vi "pco.camera_FloatingMean_Example_IMAQ.vi"() -> ()   [LabVIEW 2019]
uses:
  pco.camera/Camera.lvclass
  <vilib>/vision/NI_Vision_Development_Module.lvlib
panel:
  out "nominatorU64":u64 format="%x"
  out "denominatorU64":u64 format="%x"
  out "currentImage":T1(plugin-control)
  out "nominatorU32":u64 format="%x"
  out "denominatorU32":u64 format="%x"
  in  "averageCount":u8=10 caption="Average Count" min=2
  out "Image":T1(plugin-control)
  in  "data_format":T2(ring)=enum."Mono16"
  out "Recorded Images":u32
  in  "Quit":bool
  in  "roiY1":u64=2048 min=2 max=20000 step=1
  in  "roiX1":u64=2048 min=2 max=20000 step=1
  in  "roiY0":u64=1 min=1 max=1039 step=1
  in  "roiX0":u64=1 min=1 max=1391 step=1
  out "Image Height":u64
  out "Image Width":u64
  in  "dwImgCount":u32=10 caption="Fifo Buffer Size" max=4023
  out "Error":errorcluster {"code" format="%x"}
  # "This example shows how to compute and show a floating mean live image.\nHere the camera class is operated in fifo mode to always get next image in buffer.\nThe Average Count defines the number of images that will be averaged.\nAveraging is done by fetiching one image and using average image from previous iteration\n(avg_n = (1-1/avg_count)*avg_(n-1) + (1/avg_count)*image_n)\n\nIt is a good starting point for writing own applications.\nBut it will not be fail save, i.e. doesnt react on errors, just handles them forward to the end\n\nUsage:\nSelect your required fifo buffer size and image format and start the program.\nOnce started, the camera class will be initialized and image record will start automatically.\nInside the acquisition loop the program calculates the floating average image shows it.\nThe average count can be changed at any time.\nBy using the ROI parameters you can crop the image to select certain regions\n\nBy clicking Quit Application the record will stop and will force an exit of the camera class"
  # "pco.labview"
  # "Camera Setup"
  # "Recording Control"
  # "Parameters for image readout"
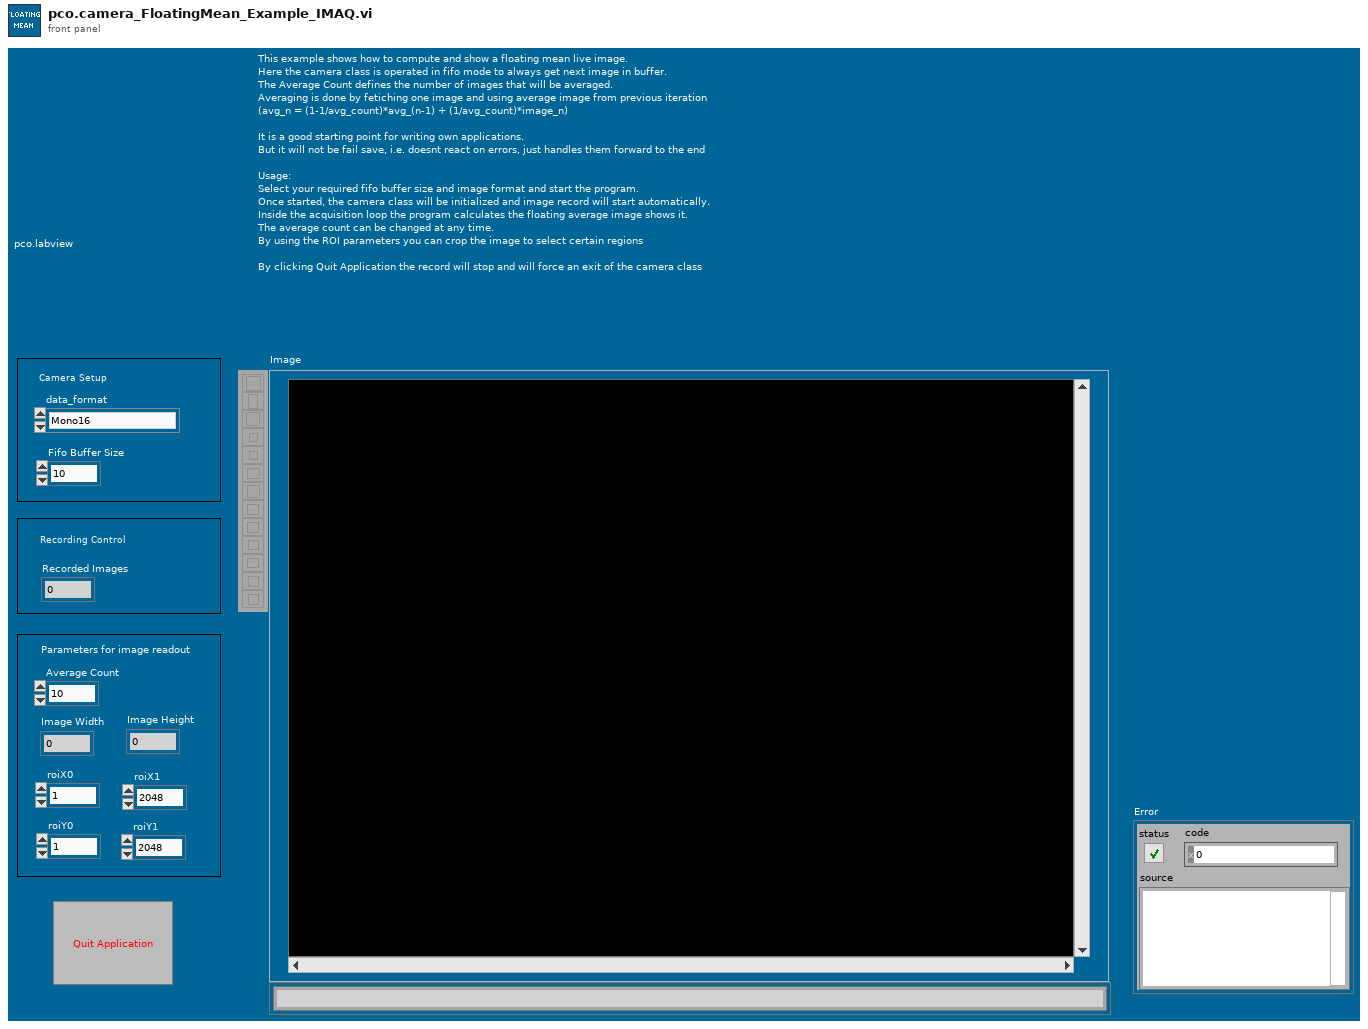
[diagram p1: front panel]
types:
  T1 = typedef "IMAQ Image.ctl" = refnum<image>
  T2 = enum16{"Undefined", "Mono8", "Mono16", "BGRA8", "RGBA8", "BGRA16", "RGBA16", "CompressedMono8"}
  T3 = enum8{"Enabled", "Disabled", "Disabled and Grayed Out"}
  T4 = enum16{"sequence", "sequence non blocking", "ring buffer", "fifo", "sequence_dpcore", "sequence_non_blocking_dpcore", "ring_buffer_dpcore", "fifo_dpcore", "tif", "multitif", "pcoraw", "b16", "dicom", "multidicom"}
  T5 = cluster{"serial":u32, "type":u16, "sub_type":u16, "interface_type":u16, "bit_resolution":u16, "min_exposure_time_s":dbl, "max_exposure_time_s":dbl, "min_exposure_step_s":dbl, "min_delay_time_s":dbl, "max_delay_time_s":dbl, "min_delay_step_s":dbl, "min_width":u64, "min_height":u64, "max_width":u64, "max_height":u64, "roi_step_horz":u64, "roi_step_vert":u64, "roi_symmetric_horz":bool, "roi_symmetric_vert":bool, "has_timestamp_mode":bool, "has_timestamp_mode_ascii_only":bool, "pixelrate_vec":u32[], "has_acquire_mode":bool, "has_ext_acquire_mode":bool, "has_metadata_mode":bool, "has_ram":bool, "binning_horz_vec":u16[], "binning_vert_vec":u16[]}
  T6 = typedef "Image Type" = u32
  T7 = typedef "Camera.lvclass/binning.ctl" = cluster{"vert":u16, "horz":u16}
  T8 = cluster{"exposure_time_s":dbl, "delay_time_s":dbl, "roi":cluster{"x0":u64, "y0":u64, "x1":u64, "y1":u64}, "timestamp_mode":u16, "pixelrate":u32, "trigger_mode":u16, "acquire_mode":u16, "metadata_mode":u16, "noisefilter_mode":u16, "binning":T7}
  T9 = cluster{"Plane 4 (alpha)":u16, "Plane 1 (Red)":u16, "Plane 2 (Green)":u16, "Plane 3 (Blue)":u16}[][]
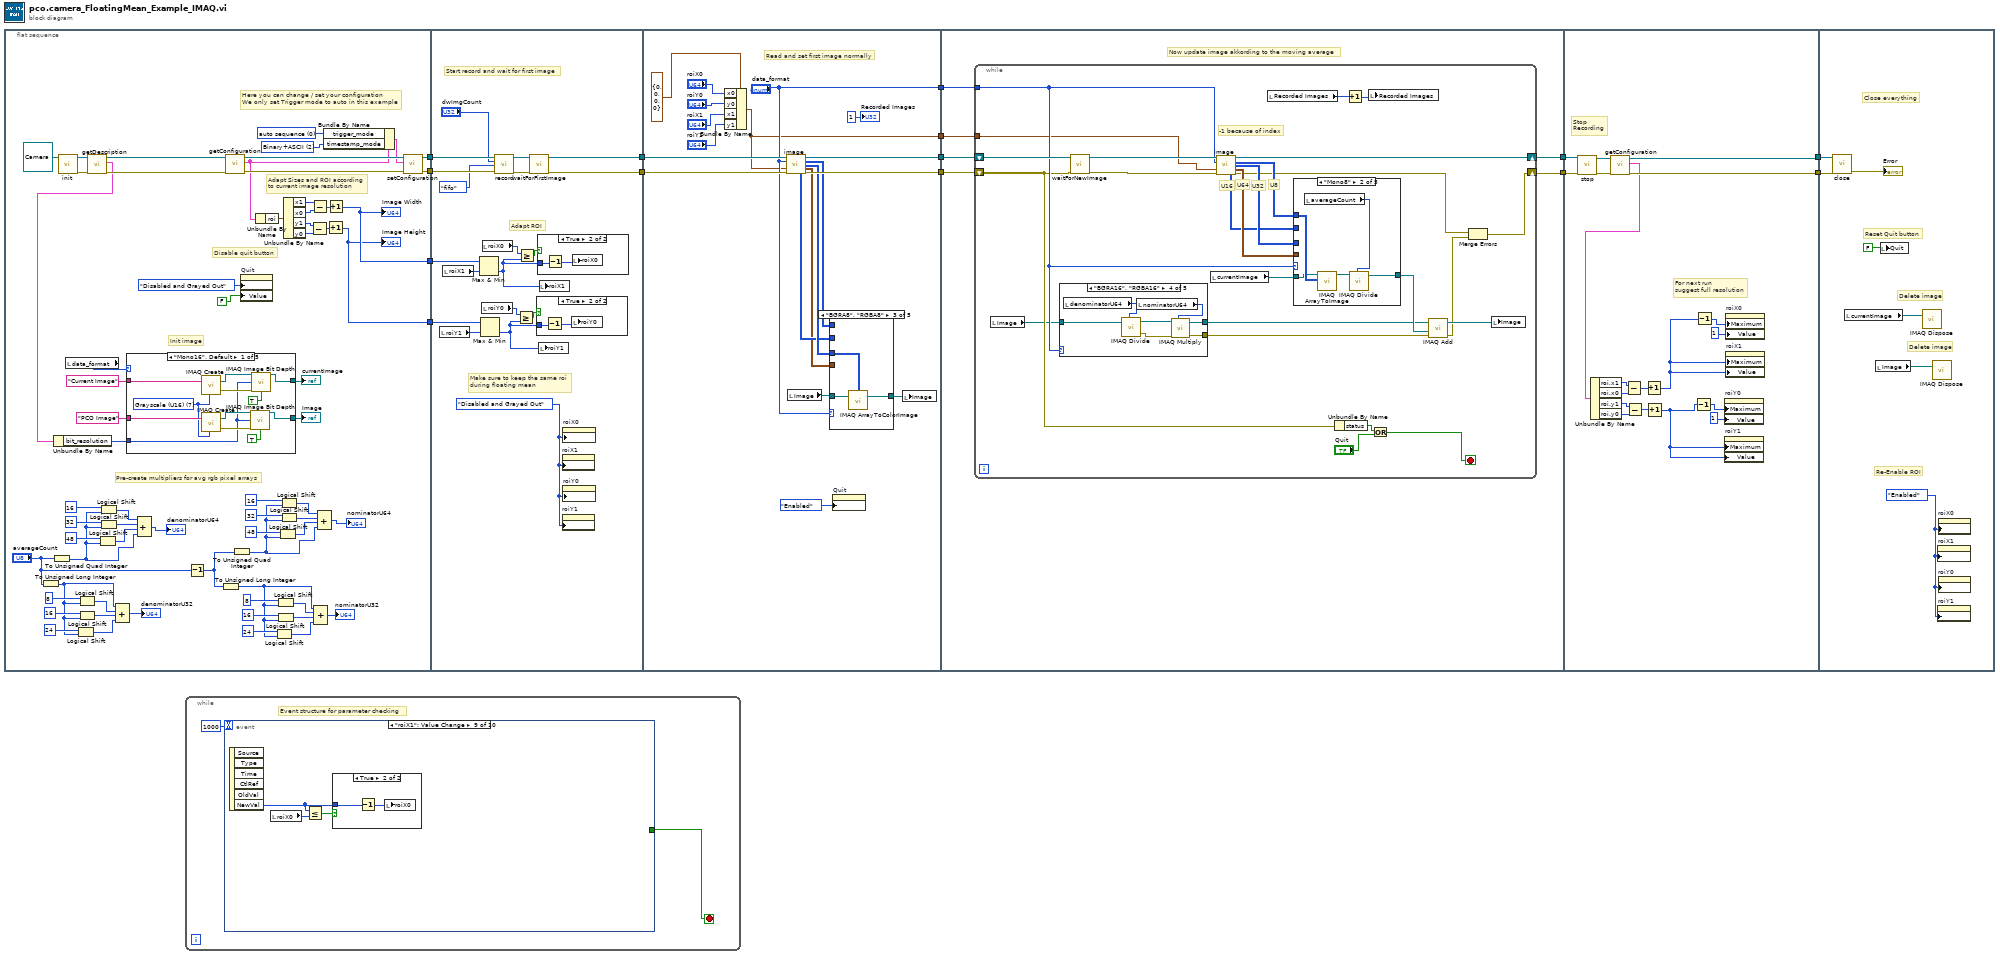
[diagram p0: block diagram]
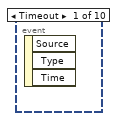
[diagram p2: hidden frame]
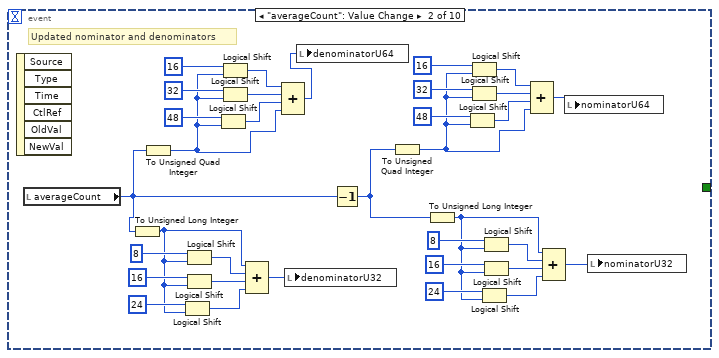
[diagram p3: hidden frame]
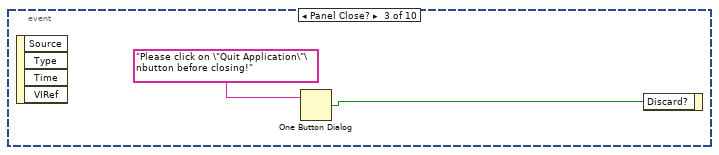
[diagram p4: hidden frame]
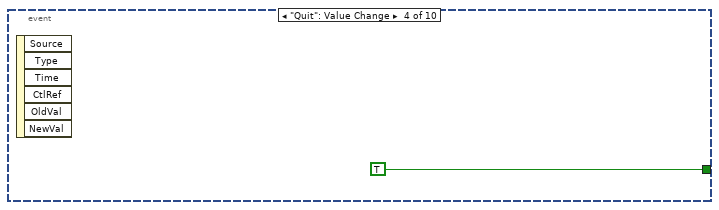
[diagram p5: hidden frame]
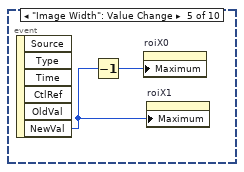
[diagram p6: hidden frame]
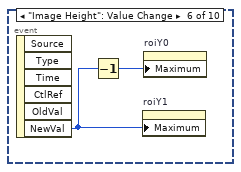
[diagram p7: hidden frame]
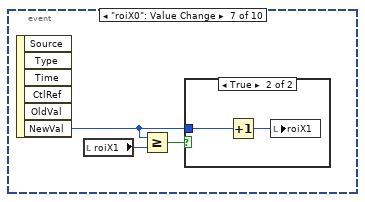
[diagram p8: hidden frame]
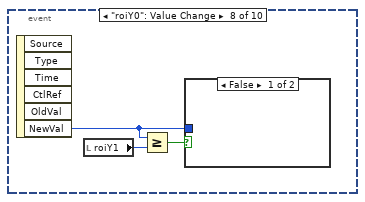
[diagram p10: hidden frame]
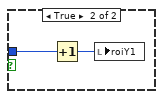
[diagram p11: hidden frame]
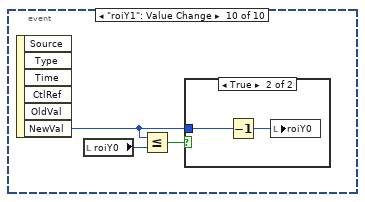
[diagram p13: hidden frame]
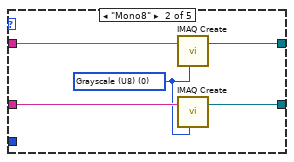
[diagram p15: hidden frame]
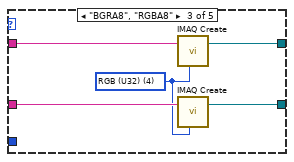
[diagram p16: hidden frame]
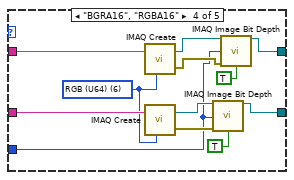
[diagram p17: hidden frame]
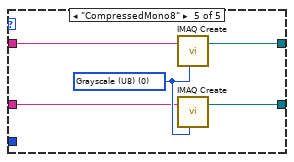
[diagram p18: hidden frame]
diagram:
  n1 = flat-sequence {
    tunnel: [w74] -> w14
    tunnel: [w73] -> w13
    tunnel: [w22] -> w2
    tunnel: [w21] -> w1
    tunnel: w14 -> [w137]
    tunnel: w13 -> [w136]
    tunnel: [w131] -> w12
    tunnel: [w130] -> w11
    tunnel: w2 -> [w127]
    tunnel: w1 -> [w125]
    tunnel: w12 -> [w159]
    tunnel: w11 -> [w158]
    tunnel: [w154] -> w10
    tunnel: [w155] -> w9
    tunnel: ["data_format"] -> w4
    tunnel: [w142] -> w3
    tunnel: w10 -> [w180]
    tunnel: w9 -> [w181]
    tunnel: [w179] -> w8
    tunnel: [w178] -> w6
    tunnel: w4 -> [w177]
    tunnel: w3 -> [w176]
    tunnel: w8 -> [w285]
    tunnel: [w280] -> w7
    tunnel: w6 -> [w284]
    tunnel: [w281] -> w5
    tunnel: w7 -> [w290]
    tunnel: w5 -> [w289]
    frame #0 {
      w64 = u16 2 items=["OFF", "Binary", "Binary+ASCII", "ASCII"] ("TimestampMode")
      w78 = u16 0 items=["auto sequence"=0, "software trigger"=1, "external exposure start & software trigger"=2, "external exposure control"=3, "external synchronized"=4, "fast external exposure control"=5, "external CDS control"=6, "slow external exposure control"=7, "external synchronized HDSDI"=258] ("TriggerMode")
      # "Pre-create multipliers for avg rgb pixel arrays"
      # "Init image"
      # "Adapt Sizes and ROI according\nto current image resolution"
      # "Disable quit button"
      # "Here you can change / set your configuration\nWe only set Trigger mode to auto in this example"
      n2 = To Unsigned Long Integer(number="averageCount") -> (unsigned 32bit integer=w44:u32)
      n3 = To Unsigned Quad Integer(1:"averageCount") -> (0:w24:u64)
      n4 = call-dynamic "init.vi"("Camera in"=refnum<class "Camera.lvclass"> refnum ("PCOCamera in")) -> ("Camera out"=w19:refnum<class "Camera.lvclass">, "error out"=w20:errorcluster)  [unwired: 8 in]
      n5 = local read "data_format"() -> (w61:T2)
      n6 = Logical Shift(y=u32 24, x=w44) -> (x << y=w55:u32)
      n7 = Logical Shift(y=u32 8, x=w44) -> (x << y=w53:u32)
      n8 = Logical Shift(y=u32 16, x=w44) -> (x << y=w54:u32)
      n9 = call-dynamic "getDescription.vi"("error in (no error)"=w20, "Camera in"=w19) -> ("error out"=w17:errorcluster, "description"=w16:T5, "Camera out"=w18:refnum<class "Camera.lvclass">)  [unwired: 7 in]
      n10 = Unbundle By Name(w16) -> ("bit_resolution"=w15:u16)
      n11 = Logical Shift(y=u32 48, x=w24) -> (x << y=w37:u64)
      n12 = Logical Shift(y=u32 16, x=w24) -> (x << y=w35:u64)
      n13 = Logical Shift(y=u32 32, x=w24) -> (x << y=w36:u64)
      n14 = Compound Arithmetic op=ADD(w44, w53, w54, w55) -> (→"denominatorU32":u32)
      n15 = case shown="\"Mono16\", Default" w61 {
        tunnel: "PCO Image" ("Image Name") -> [w91 w94 w99 w113 w116]
        tunnel: [w85 w96 w101 w107 w118] -> w60
        tunnel: [w81 w95 w100 w104 w115] -> w42
        tunnel: "Current Image" ("Image Name") -> [w89 w93 w97 w111 w114]
        tunnel: w15 -> [w80 _ _ w102 _]
        frame "Mono16", Default {
          w90 = T6 7 items=["Grayscale (U8)", "Grayscale (I16)", "Grayscale (SGL)", "Complex (CSG)", "RGB (U32)", "HSL (U32)", "RGB (U64)", "Grayscale (U16)"] ("Image Type")
          n16 = call "IMAQ Create"("Image Name"=w89, "Image Type"=w90) -> ("New Image"=w83:T1, "error out"=w82:errorcluster)  [unwired: 3 in]
          n17 = call "IMAQ Create"("Image Name"=w91, "Image Type"=w90) -> ("New Image"=w87:T1, "error out"=w86:errorcluster)  [unwired: 3 in]
          n18 = call "IMAQ Image Bit Depth"("Image"=w87, "Bit Depth (0)"=w80, "error in (no error)"=w86, "Get/Set Bit Depth? (Set)"=TRUE) -> ("Image Out"=w85:T1)  [unwired: 9 in, 2 out]
          n19 = call "IMAQ Image Bit Depth"("Image"=w83, "Bit Depth (0)"=w80, "error in (no error)"=w82, "Get/Set Bit Depth? (Set)"=TRUE) -> ("Image Out"=w81:T1)  [unwired: 9 in, 2 out]
        }
        frame "Mono8" {
          w92 = T6 0 items=["Grayscale (U8)", "Grayscale (I16)", "Grayscale (SGL)", "Complex (CSG)", "RGB (U32)", "HSL (U32)", "RGB (U64)", "Grayscale (U16)"] ("Image Type")
          n20 = call "IMAQ Create"("Image Name"=w93, "Image Type"=w92) -> ("New Image"=w95:T1)  [unwired: 3 in, 1 out]
          n21 = call "IMAQ Create"("Image Name"=w94, "Image Type"=w92) -> ("New Image"=w96:T1)  [unwired: 3 in, 1 out]
        }
        frame "BGRA8", "RGBA8" {
          w98 = T6 4 items=["Grayscale (U8)", "Grayscale (I16)", "Grayscale (SGL)", "Complex (CSG)", "RGB (U32)", "HSL (U32)", "RGB (U64)", "Grayscale (U16)"] ("Image Type")
          n22 = call "IMAQ Create"("Image Name"=w97, "Image Type"=w98) -> ("New Image"=w100:T1)  [unwired: 3 in, 1 out]
          n23 = call "IMAQ Create"("Image Name"=w99, "Image Type"=w98) -> ("New Image"=w101:T1)  [unwired: 3 in, 1 out]
        }
        frame "BGRA16", "RGBA16" {
          w112 = T6 6 items=["Grayscale (U8)", "Grayscale (I16)", "Grayscale (SGL)", "Complex (CSG)", "RGB (U32)", "HSL (U32)", "RGB (U64)", "Grayscale (U16)"] ("Image Type")
          n24 = call "IMAQ Create"("Image Name"=w111, "Image Type"=w112) -> ("New Image"=w105:T1, "error out"=w103:errorcluster)  [unwired: 3 in]
          n25 = call "IMAQ Create"("Image Name"=w113, "Image Type"=w112) -> ("New Image"=w109:T1, "error out"=w108:errorcluster)  [unwired: 3 in]
          n26 = call "IMAQ Image Bit Depth"("Image"=w109, "Bit Depth (0)"=w102, "error in (no error)"=w108, "Get/Set Bit Depth? (Set)"=TRUE) -> ("Image Out"=w107:T1)  [unwired: 9 in, 2 out]
          n27 = call "IMAQ Image Bit Depth"("Image"=w105, "Bit Depth (0)"=w102, "error in (no error)"=w103, "Get/Set Bit Depth? (Set)"=TRUE) -> ("Image Out"=w104:T1)  [unwired: 9 in, 2 out]
        }
        frame "CompressedMono8" {
          w117 = T6 0 items=["Grayscale (U8)", "Grayscale (I16)", "Grayscale (SGL)", "Complex (CSG)", "RGB (U32)", "HSL (U32)", "RGB (U64)", "Grayscale (U16)"] ("Image Type")
          n28 = call "IMAQ Create"("Image Name"=w114, "Image Type"=w117) -> ("New Image"=w115:T1)  [unwired: 3 in, 1 out]
          n29 = call "IMAQ Create"("Image Name"=w116, "Image Type"=w117) -> ("New Image"=w118:T1)  [unwired: 3 in, 1 out]
        }
      }
      "Image" <- w60
      "currentImage" <- w42
      n30 = Compound Arithmetic op=ADD(w35, w36, w37, w24) -> (→"denominatorU64":u64)
      n31 = Decrement(x="averageCount") -> (x-1=w25:u8)
      n32 = To Unsigned Long Integer(number=w25) -> (unsigned 32bit integer=w43:u32)
      n33 = call-dynamic "getConfiguration.vi"("error in (no error)"=w17, "Camera in"=w18) -> ("error out"=w76:errorcluster, "configuration"=w72:T8, "Camera out"=w77:refnum<class "Camera.lvclass">)  [unwired: 7 in]
      n34 = To Unsigned Quad Integer(1:w25) -> (0:w23:u64)
      n35 = property on="Quit" class="Bool (strict)"("DisabledEnum"=T3."Disabled and Grayed Out" ("Disabled"), "Value"=FALSE ("Stop")) -> ()  [unwired: 2 in, 2 out]
      n36 = Unbundle By Name(w72) -> ("roi"=w71:cluster{"x0":u64, "y0":u64, "x1":u64, "y1":u64})
      n37 = Logical Shift(y=u32 24, x=w43) -> (x << y=w48:u32)
      n38 = Logical Shift(y=u32 8, x=w43) -> (x << y=w46:u32)
      n39 = Logical Shift(y=u32 16, x=w43) -> (x << y=w47:u32)
      n40 = Logical Shift(y=u32 48, x=w23) -> (x << y=w29:u64)
      n41 = Logical Shift(y=u32 16, x=w23) -> (x << y=w31:u64)
      n42 = Logical Shift(y=u32 32, x=w23) -> (x << y=w30:u64)
      n43 = Unbundle By Name(w71) -> ("x1"=w69:u64, "x0"=w70:u64, "y1"=w67:u64, "y0"=w68:u64)
      n44 = Subtract(x=w67, y=w68) -> (x-y=w65:u64)
      n45 = Subtract(x=w69, y=w70) -> (x-y=w66:u64)
      n46 = Compound Arithmetic op=ADD(w43, w46, w47, w48) -> (→"nominatorU32":u32)
      n47 = Compound Arithmetic op=ADD(w31, w30, w29, w23) -> (→"nominatorU64":u64)
      n48 = Bundle By Name(cluster=w72, "trigger_mode"=w78, "timestamp_mode"=w64) -> (w75:T8)
      n49 = Increment(x=w65) -> (x+1=w21:u64)
      "Image Height" <- w21
      n50 = Increment(x=w66) -> (x+1=w22:u64)
      "Image Width" <- w22
      n51 = call-dynamic "setConfiguration.vi"("error in (no error)"=w76, "configuration"=w75, "Camera in"=w77) -> ("error out"=w73:errorcluster, "Camera out"=w74:refnum<class "Camera.lvclass">)  [unwired: 7 in]
    }
    frame #1 {
      w129 = T3."Disabled and Grayed Out" ("Disabled")
      # "Adapt ROI"
      # "Make sure to keep the same roi\nduring floating mean"
      # "Start record and wait for first image"
      n52 = local read "roiY1"() -> (w126:u64)
      n53 = local read "roiX1"() -> (w128:u64)
      n54 = Max & Min(x=w127, y=w128) -> (min(x,y)=w122:u64)  [unwired: 1 out]
      n55 = Max & Min(x=w125, y=w126) -> (min(x,y)=w119:u64)  [unwired: 1 out]
      n56 = local read "roiY0"() -> (w120:u64)
      n57 = local read "roiX0"() -> (w124:u64)
      n58 = call-dynamic "record.vi"("Camera in"=w137, "num_images"="dwImgCount", "record_mode"=T4."fifo", "error in (no error)"=w136) -> ("Camera out"=w132:refnum<class "Camera.lvclass">, "error out"=w133:errorcluster)  [unwired: 10 in]
      n59 = Greater Or Equal?(x=w120, y=w119) -> (x >= y?=w121:bool)
      n60 = Greater Or Equal?(x=w124, y=w122) -> (x >= y?=w123:bool)
      n61 = call-dynamic "waitForFirstImage.vi"("error in (no error)"=w133, "Camera in"=w132) -> ("error out"=w130:errorcluster, "Camera out"=w131:refnum<class "Camera.lvclass">)  [unwired: 8 in]
      n62 = case shown="True" w121 {
        tunnel: w119 -> [_ w139]
        frame False {
        }
        frame True {
          n63 = Decrement(x=w139) -> (x-1=w138:u64)
          n64 = local write "roiY0"(w138) -> ()
        }
      }
      n65 = case shown="True" w123 {
        tunnel: w122 -> [_ w141]
        frame False {
        }
        frame True {
          n66 = Decrement(x=w141) -> (x-1=w140:u64)
          n67 = local write "roiX0"(w140) -> ()
        }
      }
      n68 = local write "roiY1"(w119) -> ()
      n69 = local write "roiX1"(w122) -> ()
      n70 = property on="roiX1" class="DigNum (strict)"("DisabledEnum"=w129) -> ()  [unwired: 2 in, 2 out]
      n71 = property on="roiY1" class="DigNum (strict)"("DisabledEnum"=w129) -> ()  [unwired: 2 in, 2 out]
      n72 = property on="roiX0" class="DigNum (strict)"("DisabledEnum"=w129) -> ()  [unwired: 2 in, 2 out]
      n73 = property on="roiY0" class="DigNum (strict)"("DisabledEnum"=w129) -> ()  [unwired: 2 in, 2 out]
    }
    frame #2 {
      # "Read and set first image normally"
      n74 = Bundle By Name(cluster=cluster{"x0":u64, "y0":u64, "x1":u64, "y1":u64} {"x0"=0, "y0"=0, "x1"=0, "y1"=0} ("roi"), "x0"="roiX0", "y0"="roiY0", "x1"="roiX1", "y1"="roiY1") -> (w142:cluster{"x0":u64, "y0":u64, "x1":u64, "y1":u64})
      n75 = call-dynamic "image.vi"("Camera in"=w159, "data_format"="data_format", "roi"=w142, "error in (no error)"=w158) -> ("Camera out"=w154:refnum<class "Camera.lvclass">, "image (U8)"=w152:u8[][], "image (U32)"=w151:u32[][], "image (U64)"=w149:T9, "raw_image (U16)"=w150:u16[][], "error out"=w155:errorcluster)  [unwired: 4 in, 2 out]
      n76 = local read "Image"() -> (w157:T1)
      n77 = case shown="\"BGRA8\", \"RGBA8\"" "data_format" {
        tunnel: w157 -> [w163 w166 w167 w172 w175]
        tunnel: [w161 w164 w169 w170 w174] -> w148
        tunnel: w149 -> [_ _ _ w171 _]
        tunnel: w151 -> [_ _ w168 _ _]
        tunnel: w152 -> [_ w165 _ _ w173]
        tunnel: w150 -> [w162 _ _ _ _]
        frame "Mono16", Default {
          n78 = call "IMAQ ArrayToImage"("Image Pixels (U16)"=w162, "Image"=w163) -> ("Image Out"=w161:T1)  [unwired: 8 in, 1 out]
        }
        frame "Mono8" {
          n79 = call "IMAQ ArrayToImage"("Image Pixels (U8)"=w165, "Image"=w166) -> ("Image Out"=w164:T1)  [unwired: 8 in, 1 out]
        }
        frame "BGRA8", "RGBA8" {
          n80 = call "IMAQ ArrayToColorImage"("Image Pixels (U32)"=w168, "Image"=w167) -> ("Image Out"=w169:T1)  [unwired: 3 in, 1 out]
        }
        frame "BGRA16", "RGBA16" {
          n81 = call "IMAQ ArrayToColorImage"("Image"=w172, "Image Pixels (U64)"=w171) -> ("Image Out"=w170:T1)  [unwired: 3 in, 1 out]
        }
        frame "CompressedMono8" {
          n82 = call "IMAQ ArrayToImage"("Image Pixels (U8)"=w173, "Image"=w175) -> ("Image Out"=w174:T1)  [unwired: 8 in, 1 out]
        }
      }
      n83 = property on="Quit" class="Bool (strict)"("DisabledEnum"=T3."Enabled" ("Disabled")) -> ()  [unwired: 2 in, 2 out]
      n84 = local write "Image"(w148) -> ()
      "Recorded Images" <- u32 1 ("Recorded Images")
    }
    frame #3 {
      # "Now update image akkording to the moving average"
      n85 = while {
        shift-right: [w206] -> w179
        shift-left: w180 -> [w205]
        shift-right: [w186] -> w178
        shift-left: w181 -> [w192]
        tunnel: w177 -> [w195]
        tunnel: w176 -> [w182]
        stop <- w189 stop-if-true
        # "-1 because of index"
        # "U64"
        # "U32"
        # "U16"
        # "U8"
        n86 = local read "Image"() -> (w185:T1)
        n87 = case shown="\"BGRA16\", \"RGBA16\"" w195 {
          tunnel: w185 -> [w210 w218 w226 w233 w239]
          tunnel: [w209 w216 w223 w232 w237] -> w183
          tunnel: [w207 w214 w221 w230 w235] -> w193
          frame "Mono16", Default {
            n88 = local read "averageCount"() -> (w212:u8)
            n89 = call "IMAQ Divide"("Image Src A"=w210, "Constant"=w212) -> ("Image Dst Out"=w213:T1, "error out"=w208:errorcluster)  [unwired: 5 in]
            n90 = Decrement(x=w212) -> (x-1=w211:u8)
            n91 = call "IMAQ Multiply"("Image Src A"=w213, "Constant"=w211, "error in (no error)"=w208) -> ("Image Dst Out"=w209:T1, "error out"=w207:errorcluster)  [unwired: 4 in]
          }
          frame "Mono8" {
            n92 = local read "averageCount"() -> (w217:u8)
            n93 = call "IMAQ Divide"("Image Src A"=w218, "Constant"=w217) -> ("Image Dst Out"=w220:T1, "error out"=w215:errorcluster)  [unwired: 5 in]
            n94 = Decrement(x=w217) -> (x-1=w219:u8)
            n95 = call "IMAQ Multiply"("Image Src A"=w220, "Constant"=w219, "error in (no error)"=w215) -> ("Image Dst Out"=w216:T1, "error out"=w214:errorcluster)  [unwired: 4 in]
          }
          frame "BGRA8", "RGBA8" {
            n96 = local read "denominatorU32"() -> (w225:u64)
            n97 = call "IMAQ Divide"("Image Src A"=w226, "Constant"=w225) -> ("Image Dst Out"=w227:T1, "error out"=w222:errorcluster)  [unwired: 5 in]
            n98 = local read "nominatorU32"() -> (w224:u64)
            n99 = call "IMAQ Multiply"("Image Src A"=w227, "Constant"=w224, "error in (no error)"=w222) -> ("Image Dst Out"=w223:T1, "error out"=w221:errorcluster)  [unwired: 4 in]
          }
          frame "BGRA16", "RGBA16" {
            n100 = local read "denominatorU64"() -> (w229:u64)
            n101 = call "IMAQ Divide"("Image Src A"=w233, "Constant"=w229) -> ("Image Dst Out"=w234:T1, "error out"=w231:errorcluster)  [unwired: 5 in]
            n102 = local read "nominatorU64"() -> (w228:u64)
            n103 = call "IMAQ Multiply"("Image Src A"=w234, "Constant"=w228, "error in (no error)"=w231) -> ("Image Dst Out"=w232:T1, "error out"=w230:errorcluster)  [unwired: 4 in]
          }
          frame "CompressedMono8" {
            n104 = local read "averageCount"() -> (w238:u8)
            n105 = call "IMAQ Divide"("Image Src A"=w239, "Constant"=w238) -> ("Image Dst Out"=w241:T1, "error out"=w236:errorcluster)  [unwired: 5 in]
            n106 = Decrement(x=w238) -> (x-1=w240:u8)
            n107 = call "IMAQ Multiply"("Image Src A"=w241, "Constant"=w240, "error in (no error)"=w236) -> ("Image Dst Out"=w237:T1, "error out"=w235:errorcluster)  [unwired: 4 in]
          }
        }
        n108 = call-dynamic "waitForNewImage.vi"("error in (no error)"=w192, "Camera in"=w205) -> ("error out"=w201:errorcluster, "Camera out"=w202:refnum<class "Camera.lvclass">)  [unwired: 8 in]
        n109 = local read "currentImage"() -> (w194:T1)
        n110 = call-dynamic "image.vi"("Camera in"=w202, "data_format"=w195, "roi"=w182, "error in (no error)"=w201) -> ("Camera out"=w206:refnum<class "Camera.lvclass">, "image (U8)"=w200:u8[][], "image (U32)"=w198:u32[][], "image (U64)"=w199:T9, "raw_image (U16)"=w197:u16[][], "error out"=w187:errorcluster)  [unwired: 4 in, 2 out]
        n111 = local read "Recorded Images"() -> (w204:u32)
        n112 = case shown="\"Mono8\"" w195 {
          tunnel: [w243 w249 w254 w259 w263] -> w184
          tunnel: w199 -> [_ _ _ w261 _]
          tunnel: w198 -> [_ _ w256 _ _]
          tunnel: w200 -> [_ w251 _ _ w266]
          tunnel: w197 -> [w246 _ _ _ _]
          tunnel: w194 -> [w242 w247 w252 w257 w262]
          frame "Mono16", Default {
            n113 = local read "averageCount"() -> (w244:u8)
            n114 = call "IMAQ ArrayToImage"("Image Pixels (U16)"=w246, "Image"=w242) -> ("Image Out"=w245:T1)  [unwired: 8 in, 1 out]
            n115 = call "IMAQ Divide"("Image Src A"=w245, "Constant"=w244) -> ("Image Dst Out"=w243:T1)  [unwired: 5 in, 1 out]
          }
          frame "Mono8" {
            n116 = local read "averageCount"() -> (w248:u8)
            n117 = call "IMAQ ArrayToImage"("Image Pixels (U8)"=w251, "Image"=w247) -> ("Image Out"=w250:T1)  [unwired: 8 in, 1 out]
            n118 = call "IMAQ Divide"("Image Src A"=w250, "Constant"=w248) -> ("Image Dst Out"=w249:T1)  [unwired: 5 in, 1 out]
          }
          frame "BGRA8", "RGBA8" {
            n119 = local read "denominatorU32"() -> (w253:u64)
            n120 = call "IMAQ ArrayToColorImage"("Image Pixels (U32)"=w256, "Image"=w252) -> ("Image Out"=w255:T1)  [unwired: 3 in, 1 out]
            n121 = call "IMAQ Divide"("Image Src A"=w255, "Constant"=w253) -> ("Image Dst Out"=w254:T1)  [unwired: 5 in, 1 out]
          }
          frame "BGRA16", "RGBA16" {
            n122 = local read "denominatorU64"() -> (w258:u64)
            n123 = call "IMAQ ArrayToColorImage"("Image"=w257, "Image Pixels (U64)"=w261) -> ("Image Out"=w260:T1)  [unwired: 3 in, 1 out]
            n124 = call "IMAQ Divide"("Image Src A"=w260, "Constant"=w258) -> ("Image Dst Out"=w259:T1)  [unwired: 5 in, 1 out]
          }
          frame "CompressedMono8" {
            n125 = local read "averageCount"() -> (w264:u8)
            n126 = call "IMAQ ArrayToImage"("Image Pixels (U8)"=w266, "Image"=w262) -> ("Image Out"=w265:T1)  [unwired: 8 in, 1 out]
            n127 = call "IMAQ Divide"("Image Src A"=w265, "Constant"=w264) -> ("Image Dst Out"=w263:T1)  [unwired: 5 in, 1 out]
          }
        }
        n128 = Unbundle By Name(w192) -> ("status"=w191:bool)
        n129 = Increment(x=w204) -> (x+1=w203:u32)
        n130 = local write "Recorded Images"(w203) -> ()
        n131 = Or(x=w191, y="Quit") -> (x .or. y?=w189:bool)
        n132 = call "IMAQ Add"("Image Src A"=w183, "Image Src B"=w184, "error in (no error)"=w193) -> ("Image Dst Out"=w196:T1, "error out"=w188:errorcluster)  [unwired: 4 in]
        n133 = Merge Errors(w187, w188) -> (w186:errorcluster)
        n134 = local write "Image"(w196) -> ()
      }
    }
    frame #4 {
      # "For next run \nsuggest full resolution"
      # "Stop \nRecording"
      n135 = call-dynamic "stop.vi"("error in (no error)"=w284, "Camera in"=w285) -> ("error out"=w282:errorcluster, "Camera out"=w283:refnum<class "Camera.lvclass">)  [unwired: 8 in]
      n136 = call-dynamic "getConfiguration.vi"("error in (no error)"=w282, "Camera in"=w283) -> ("error out"=w281:errorcluster, "configuration"=w267:T8, "Camera out"=w280:refnum<class "Camera.lvclass">)  [unwired: 7 in]
      n137 = Unbundle By Name(w267) -> ("roi.x1"=w273:u64, "roi.x0"=w272:u64, "roi.y1"=w271:u64, "roi.y0"=w270:u64)
      n138 = Subtract(x=w273, y=w272) -> (x-y=w274:u64)
      n139 = Subtract(x=w271, y=w270) -> (x-y=w275:u64)
      n140 = Increment(x=w274) -> (x+1=w278:u64)
      n141 = Increment(x=w275) -> (x+1=w277:u64)
      n142 = Decrement(x=w277) -> (x-1=w276:u64)
      n143 = Decrement(x=w278) -> (x-1=w279:u64)
      n144 = property on="roiY0" class="DigNum (strict)"("Maximum"=w276, "Value"=u64 1 ("roiY0")) -> ()  [unwired: 2 in, 2 out]
      n145 = property on="roiY1" class="DigNum (strict)"("Maximum"=w277, "Value"=w277) -> ()  [unwired: 2 in, 2 out]
      n146 = property on="roiX0" class="DigNum (strict)"("Maximum"=w279, "Value"=u64 1 ("roiX0")) -> ()  [unwired: 2 in, 2 out]
      n147 = property on="roiX1" class="DigNum (strict)"("Maximum"=w278, "Value"=w278) -> ()  [unwired: 2 in, 2 out]
    }
    frame #5 {
      w286 = T3."Enabled" ("Disabled")
      # "Re-Enable ROI"
      # "Delete image"
      # "Delete image"
      # "Reset Quit button"
      # "Close everything"
      n148 = call-dynamic "close.vi"("error in (no error)"=w289, "Camera in"=w290) -> ("error out"=→"Error":errorcluster)  [unwired: 9 in]
      n149 = local read "currentImage"() -> (w287:T1)
      n150 = local read "Image"() -> (w288:T1)
      n151 = local write "Quit"(FALSE ("Stop")) -> ()
      n152 = call "IMAQ Dispose"("Image"=w287) -> ()  [unwired: 5 in, 1 out]
      n153 = call "IMAQ Dispose"("Image"=w288) -> ()  [unwired: 5 in, 1 out]
      n154 = property on="roiX1" class="DigNum (strict)"("DisabledEnum"=w286) -> ()  [unwired: 2 in, 2 out]
      n155 = property on="roiY1" class="DigNum (strict)"("DisabledEnum"=w286) -> ()  [unwired: 2 in, 2 out]
      n156 = property on="roiX0" class="DigNum (strict)"("DisabledEnum"=w286) -> ()  [unwired: 2 in, 2 out]
      n157 = property on="roiY0" class="DigNum (strict)"("DisabledEnum"=w286) -> ()  [unwired: 2 in, 2 out]
    }
  }
  n158 = while {
    stop <- w293 stop-if-true
    # "Event structure for parameter checking"
    n159 = event shown="[8] \"roiX1\": Value Change" {
      selector: _ -> [_ _ _ _ _ _ _ _ _ _]
      dyn-events: _ -> [_ _ _ _ _ _ _ _ _ _]
      timeout: 1000 -> [_ _ _ _ _ _ _ _ _ _]
      tunnel: [_ _ _ TRUE _ _ _ _ _ _] -> w293
      event Timeout {
        n160 = event-data() -> ()  [unwired: 1 in, 3 out]
      }
      event "averageCount": Value Change {
        # "Updated nominator and denominators"
        n161 = event-data() -> ()  [unwired: 1 in, 6 out]
        n162 = local read "averageCount"() -> (w301:u8)
        n163 = To Unsigned Long Integer(number=w301) -> (unsigned 32bit integer=w314:u32)
        n164 = To Unsigned Quad Integer(1:w301) -> (0:w298:u64)
        n165 = Logical Shift(y=u32 24, x=w314) -> (x << y=w325:u32)
        n166 = Logical Shift(y=u32 8, x=w314) -> (x << y=w323:u32)
        n167 = Logical Shift(y=u32 16, x=w314) -> (x << y=w324:u32)
        n168 = Logical Shift(y=u32 48, x=w298) -> (x << y=w304:u64)
        n169 = Logical Shift(y=u32 16, x=w298) -> (x << y=w306:u64)
        n170 = Logical Shift(y=u32 32, x=w298) -> (x << y=w305:u64)
        n171 = Compound Arithmetic op=ADD(w314, w323, w324, w325) -> (w316:u32)
        n172 = Compound Arithmetic op=ADD(w306, w305, w304, w298) -> (w299:u64)
        n173 = local write "denominatorU32"(w316) -> ()
        n174 = local write "denominatorU64"(w299) -> ()
        n175 = Decrement(x=w301) -> (x-1=w307:u8)
        n176 = To Unsigned Quad Integer(1:w307) -> (0:w297:u64)
        n177 = To Unsigned Long Integer(number=w307) -> (unsigned 32bit integer=w313:u32)
        n178 = Logical Shift(y=u32 48, x=w297) -> (x << y=w310:u64)
        n179 = Logical Shift(y=u32 16, x=w297) -> (x << y=w312:u64)
        n180 = Logical Shift(y=u32 32, x=w297) -> (x << y=w311:u64)
        n181 = Logical Shift(y=u32 24, x=w313) -> (x << y=w319:u32)
        n182 = Logical Shift(y=u32 8, x=w313) -> (x << y=w317:u32)
        n183 = Logical Shift(y=u32 16, x=w313) -> (x << y=w318:u32)
        n184 = Compound Arithmetic op=ADD(w312, w311, w310, w297) -> (w300:u64)
        n185 = Compound Arithmetic op=ADD(w313, w317, w318, w319) -> (w315:u32)
        n186 = local write "nominatorU64"(w300) -> ()
        n187 = local write "nominatorU32"(w315) -> ()
      }
      event Panel Close? {
        n188 = event-data() -> ()  [unwired: 1 in, 4 out]
        n189 = One Button Dialog(message="Please click on \"Quit Application\"\nbutton before closing!") -> (true=w329:bool)  [unwired: 1 in]
        n190 = event-data("Discard?"=w329) -> ()  [unwired: 1 in, 1 out]
      }
      event "Quit": Value Change {
        n191 = event-data() -> ()  [unwired: 1 in, 6 out]
      }
      event "Image Width": Value Change {
        n192 = event-data() -> ("NewVal"=w332:u64)  [unwired: 1 in, 5 out]
        n193 = Decrement(x=w332) -> (x-1=w333:u64)
        n194 = property on="roiX0" class="DigNum (strict)"("Maximum"=w333) -> ()  [unwired: 2 in, 2 out]
        n195 = property on="roiX1" class="DigNum (strict)"("Maximum"=w332) -> ()  [unwired: 2 in, 2 out]
      }
      event "Image Height": Value Change {
        n196 = event-data() -> ("NewVal"=w334:u64)  [unwired: 1 in, 5 out]
        n197 = Decrement(x=w334) -> (x-1=w335:u64)
        n198 = property on="roiY1" class="DigNum (strict)"("Maximum"=w334) -> ()  [unwired: 2 in, 2 out]
        n199 = property on="roiY0" class="DigNum (strict)"("Maximum"=w335) -> ()  [unwired: 2 in, 2 out]
      }
      event "roiX0": Value Change {
        n200 = event-data() -> ("NewVal"=w336:u64)  [unwired: 1 in, 5 out]
        n201 = local read "roiX1"() -> (w338:u64)
        n202 = Greater Or Equal?(x=w336, y=w338) -> (x >= y?=w337:bool)
        n203 = case shown="True" w337 {
          tunnel: w336 -> [_ w340]
          frame False {
          }
          frame True {
            n204 = Increment(x=w340) -> (x+1=w339:u64)
            n205 = local write "roiX1"(w339) -> ()
          }
        }
      }
      event "roiY0": Value Change {
        n206 = event-data() -> ("NewVal"=w341:u64)  [unwired: 1 in, 5 out]
        n207 = local read "roiY1"() -> (w343:u64)
        n208 = Greater Or Equal?(x=w341, y=w343) -> (x >= y?=w342:bool)
        n209 = case shown="False" w342 {
          tunnel: w341 -> [_ w345]
          frame False {
          }
          frame True {
            n210 = Increment(x=w345) -> (x+1=w344:u64)
            n211 = local write "roiY1"(w344) -> ()
          }
        }
      }
      event "roiX1": Value Change {
        n212 = event-data() -> ("NewVal"=w346:u64)  [unwired: 1 in, 5 out]
        n213 = local read "roiX0"() -> (w348:u64)
        n214 = Less Or Equal?(x=w346, y=w348) -> (x <= y?=w347:bool)
        n215 = case shown="True" w347 {
          tunnel: w346 -> [_ w350]
          frame False {
          }
          frame True {
            n216 = Decrement(x=w350) -> (x-1=w349:u64)
            n217 = local write "roiX0"(w349) -> ()
          }
        }
      }
      event "roiY1": Value Change {
        n218 = event-data() -> ("NewVal"=w351:u64)  [unwired: 1 in, 5 out]
        n219 = local read "roiY0"() -> (w353:u64)
        n220 = Less Or Equal?(x=w351, y=w353) -> (x <= y?=w352:bool)
        n221 = case shown="True" w352 {
          tunnel: w351 -> [_ w355]
          frame False {
          }
          frame True {
            n222 = Decrement(x=w355) -> (x-1=w354:u64)
            n223 = local write "roiY0"(w354) -> ()
          }
        }
      }
    }
  }
